vi "Discretization_DiscretizeAB.vi"(6 "dT_Seconds":dbl, 8 "ContB":T1, 9 "ContA":T1, 10 "Inputs":i32, 11 "States":i32) -> (0 "Error":bool, 1 "DiscB":T1, 3 "DiscA":T1)   [LabVIEW 2019, in "Trajectory_Library.lvlib"]
doc: "Discretizes the given continuous A and B matrices.\n \nInputs:\n - States -- Nat representing the states of the system.\n - Inputs -- Nat representing the inputs to the system.\n - contA -- Continuous system matrix.\n - contB -- Continuous input matrix.\n - dtSeconds -- Discretization timestep.\n\nOutputs:\n - discA -- Discretized A matrix\n - discB -- Discretized B matrix\n - error -- If TRUE, an error occured."
uses:
  Trajectory_Library.lvlib
  <vilib>/Analysis/Matrix/Datatypes/RealMatrix.ctl
  <vilib>/Analysis/Matrix/Numeric/Multiply/Multiply - RM,R.vi
  <vilib>/Analysis/Matrix/NI_Matrix.lvlib
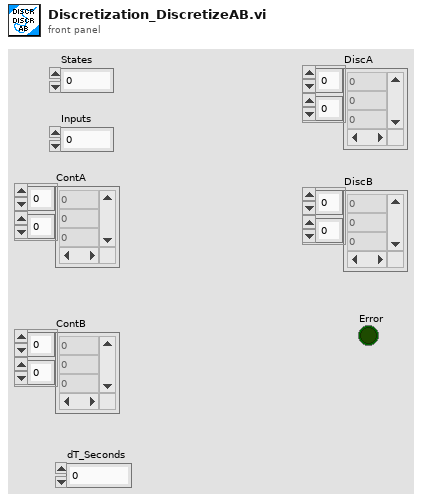
[diagram p1: front panel]
types:
  T1 = typedef "NI_Matrix.lvlib/RealMatrix.ctl" = dbl[][]
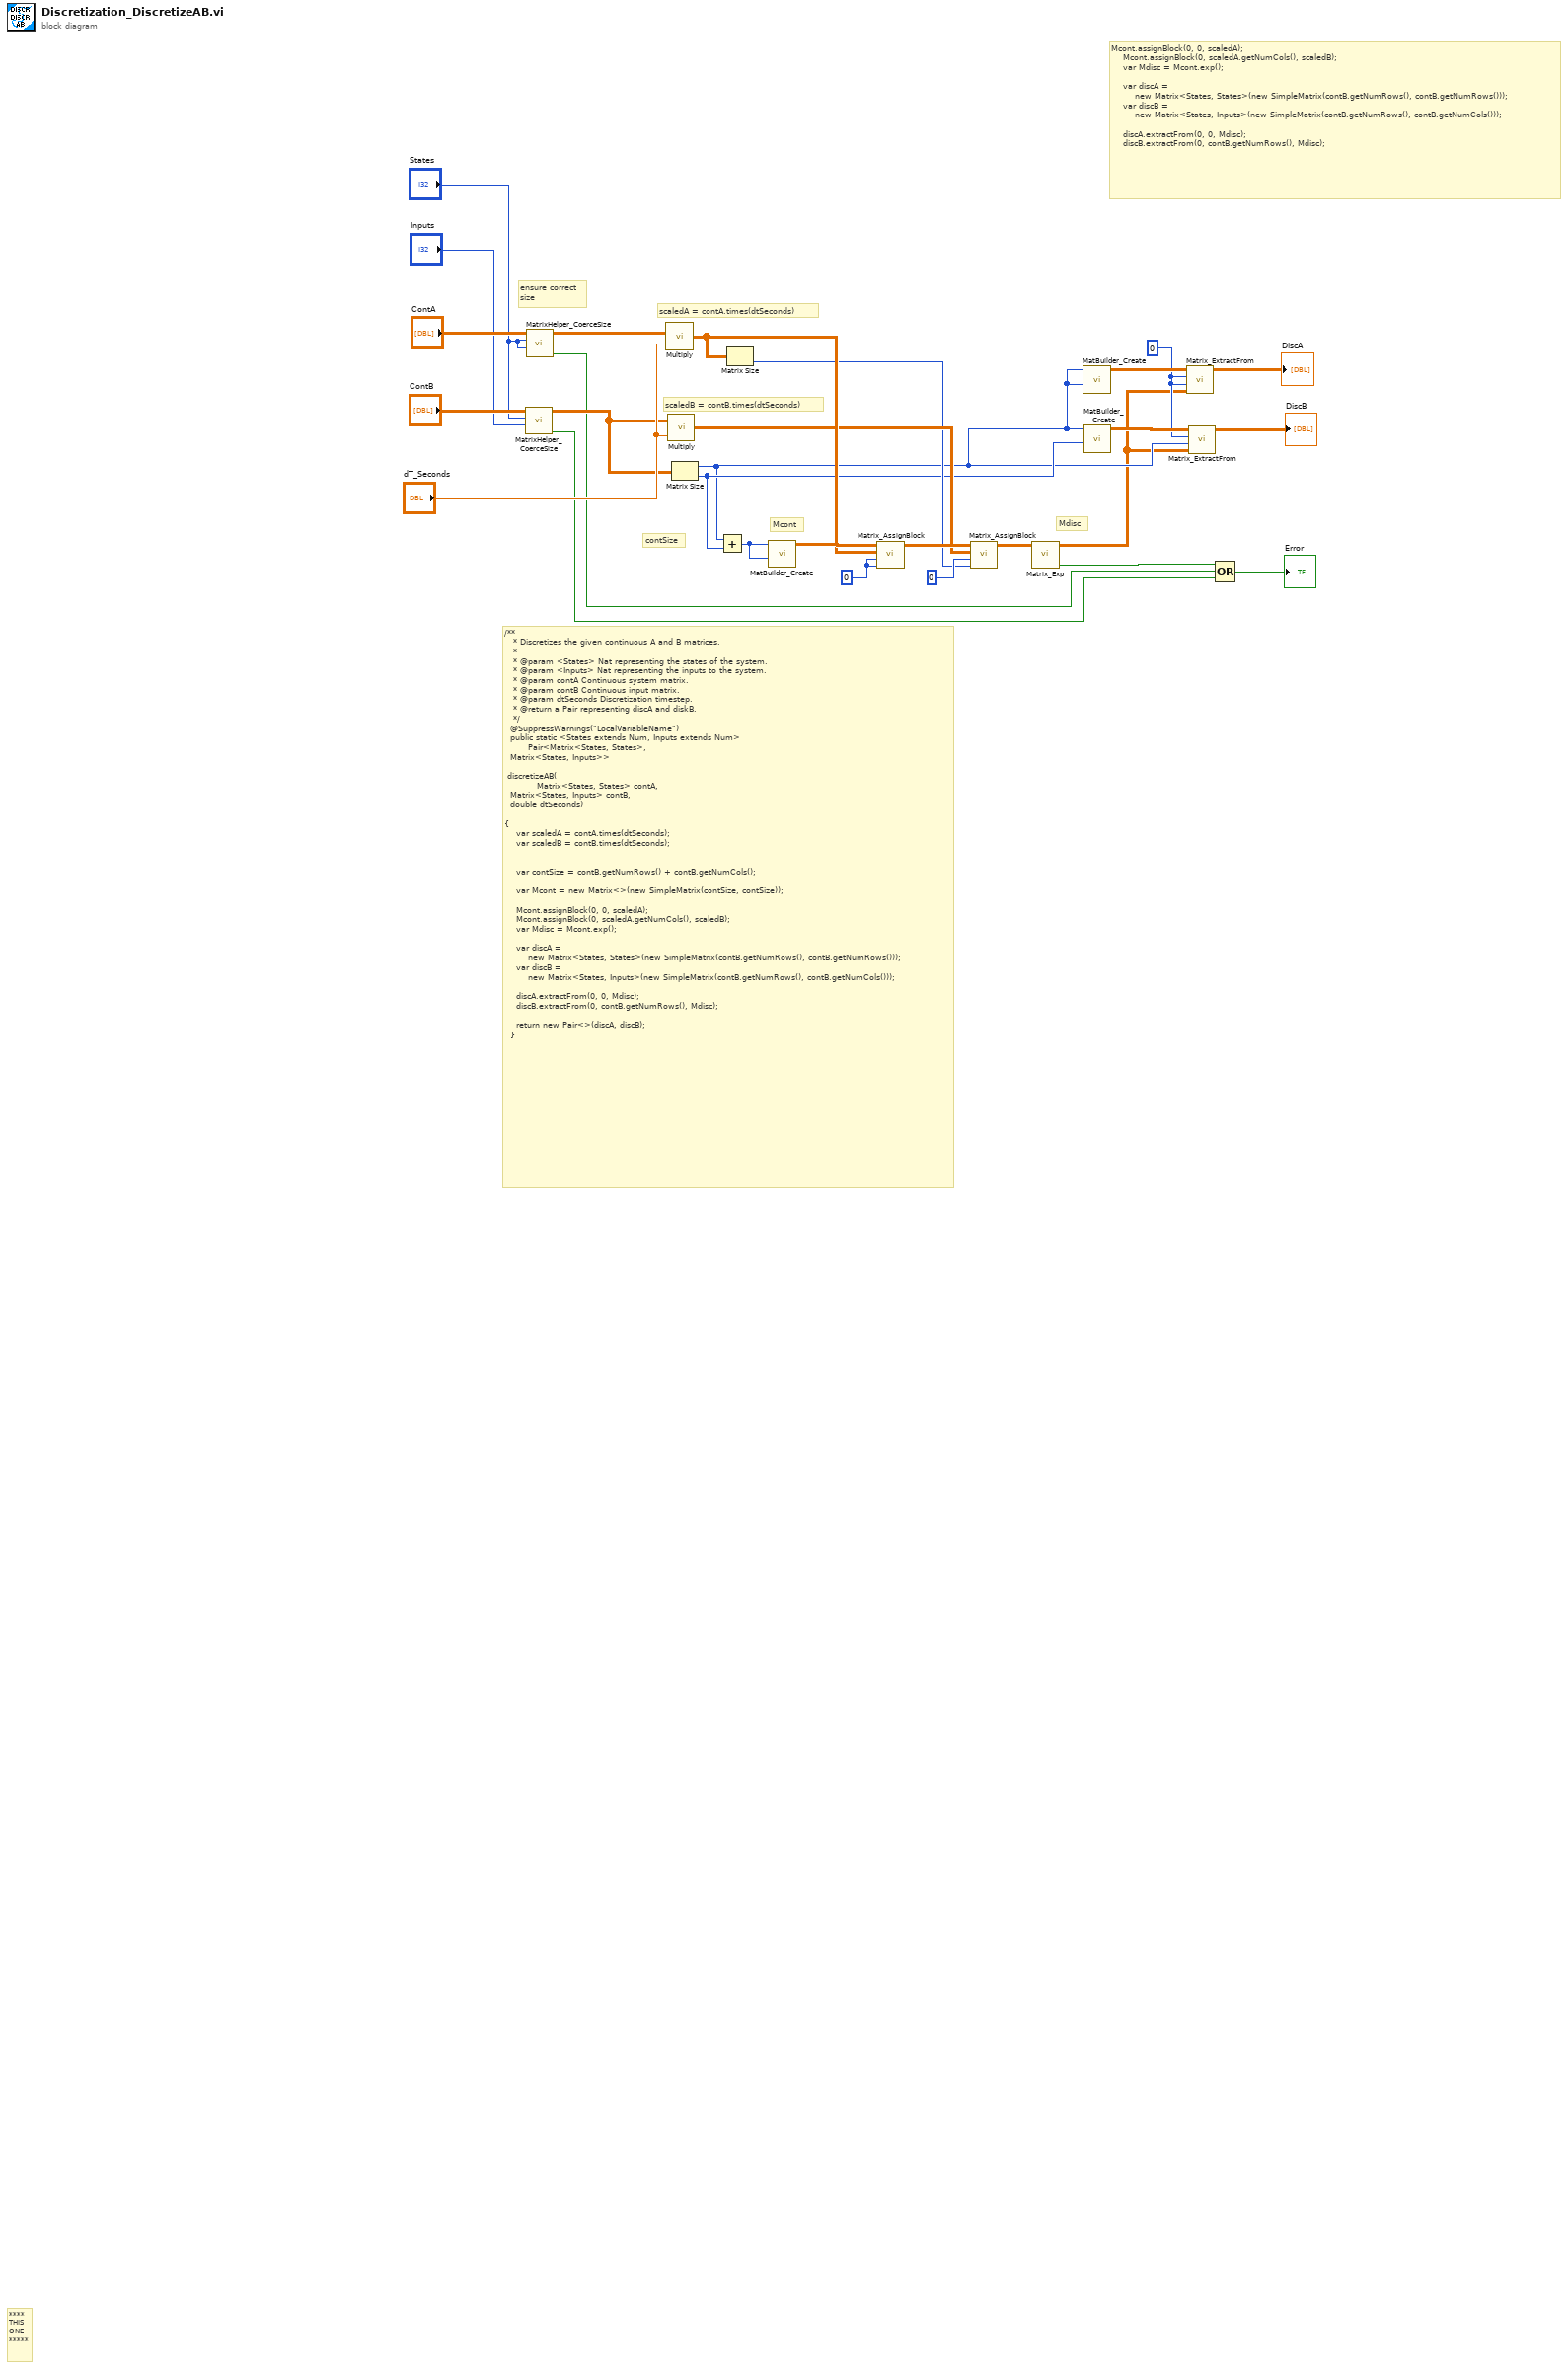
[diagram p0: block diagram]
diagram:
  w9 = 0 ("StartingRow")
  w18 = 0 ("disabled index (row)")
  # "Mcont.assignBlock(0, 0, scaledA);\n    Mcont.assignBlock(0, scaledA.getNumCols(), scaledB);\n    var Mdisc = Mcont.exp();\n\n    var discA =\n        new Matrix<States, States>(new SimpleMatrix(contB.getNumRows(), contB.getNumRows()));\n    var discB =\n        new Matrix<States, Inputs>(new SimpleMatrix(contB.getNumRows(), contB.getNumCols()));\n\n    discA.extractFrom(0, 0, Mdisc);\n    discB.extractFrom(0, contB.getNumRows(), Mdisc);"
  # "Mdisc"
  # "Mcont"
  # "contSize"
  # "scaledB = contB.times(dtSeconds)"
  # "scaledA = contA.times(dtSeconds)"
  # "ensure correct\nsize"
  # "/**\n   * Discretizes the given continuous A and B matrices.\n   *\n   * @param <States> Nat representing the states of the system.\n   * @param <Inputs> Nat representing the inputs to the system.\n   * @param contA Continuous system matrix.\n   * @param contB Continuous input matrix.\n   * @param dtSeconds Discretization timestep.\n   * @return a Pair representing discA and diskB.\n   */\n  @SuppressWarnings(\"LocalVariableName\")\n  public static <States extends Num, Inputs extends Num>\n      \t\tPair<Matrix<States, States>, \n\t\tMatrix<States, Inputs>> \n\n\tdiscretizeAB(\n          \tMatrix<States, States> contA, \n\t\tMatrix<States, Inputs> contB, \n\t\tdouble dtSeconds) \n\n{\n    var scaledA = contA.times(dtSeconds);\n    var scaledB = contB.times(dtSeconds);\n\n\n    var contSize = contB.getNumRows() + contB.getNumCols();\n\n    var Mcont = new Matrix<>(new SimpleMatrix(contSize, contSize));\n\n    Mcont.assignBlock(0, 0, scaledA);\n    Mcont.assignBlock(0, scaledA.getNumCols(), scaledB);\n    var Mdisc = Mcont.exp();\n\n    var discA =\n        new Matrix<States, States>(new SimpleMatrix(contB.getNumRows(), contB.getNumRows()));\n    var discB =\n        new Matrix<States, Inputs>(new SimpleMatrix(contB.getNumRows(), contB.getNumCols()));\n\n    discA.extractFrom(0, 0, Mdisc);\n    discB.extractFrom(0, contB.getNumRows(), Mdisc);\n\n    return new Pair<>(discA, discB);\n  }"
  # "****\nTHIS\nONE\n*****"
  n1 = call "MatrixHelper_CoerceSize.vi"("Columns"="Inputs", "Rows"="States", "input matrix"="ContB") -> ("Coerced"=w2:bool, "output matrix"=w23:T1)  [unwired: 7 in]
  n2 = call "MatrixHelper_CoerceSize.vi"("Columns"="States", "Rows"="States", "input matrix"="ContA") -> ("Coerced"=w3:bool, "output matrix"=w27:T1)  [unwired: 7 in]
  n3 = call-poly <vilib>:"Multiply.vi"("Real Scalar c"="dT_Seconds", "Real Matrix A"=w27) -> ("A * c"=w19:T1)
  n4 = call-poly <vilib>:"Multiply.vi"("Real Scalar c"="dT_Seconds", "Real Matrix A"=w23) -> ("A * c"=w15:T1)
  n5 = Matrix Size(0:w23) -> (1:w8:i32, 2:w12:i32)
  n6 = Add(x=w8, y=w12) -> (x+y=w25:i32)
  n7 = Matrix Size(0:w19) -> (2:w13:i32)  [unwired: 1 out]
  n8 = call "MatBuilder_Create.vi"("Columns"=w25, "Rows"=w25) -> ("output matrix"=w20:T1)  [unwired: 9 in]
  n9 = call "Matrix_AssignBlock.vi"("StartColumn"=w18, "StartRow"=w18, "Other Matrix"=w19, "input matrix"=w20) -> ("output matrix"=w16:T1)  [unwired: 7 in]
  n10 = call "Matrix_AssignBlock.vi"("StartColumn"=w13, "StartRow"=0 ("disabled index (row)"), "Other Matrix"=w15, "input matrix"=w16) -> ("output matrix"=w17:T1)  [unwired: 7 in]
  n11 = call "Matrix_Exp.vi"("input matrix"=w17) -> ("Error"=w4:bool, "output matrix"=w7:T1)  [unwired: 9 in]
  n12 = call "MatBuilder_Create.vi"("Columns"=w8, "Rows"=w8) -> ("output matrix"=w11:T1)  [unwired: 9 in]
  n13 = call "MatBuilder_Create.vi"("Columns"=w12, "Rows"=w8) -> ("output matrix"=w10:T1)  [unwired: 9 in]
  n14 = call "Matrix_ExtractFrom.vi"("other"=w7, "StartingColumn"=w9, "StartingRow"=w9, "input matrix"=w11) -> ("output column"=→"DiscA":T1)  [unwired: 7 in]
  n15 = call "Matrix_ExtractFrom.vi"("other"=w7, "StartingColumn"=w8, "StartingRow"=w9, "input matrix"=w10) -> ("output column"=→"DiscB":T1)  [unwired: 7 in]
  n16 = Compound Arithmetic op=OR(w4, w3, w2) -> (→"Error":bool)
